vi "mxwScript_Cmnd2Str_startGeneration.vi"(8 "error in (no error)":errorcluster, 11 "data":variant) -> (0 "error out":errorcluster, 3 "outputString":string)   [LabVIEW 2020]
uses:
  codeGenAPISupport.llb/cgAPI_mxwScript_Cmnd_StartGenerationCommandData.ctl
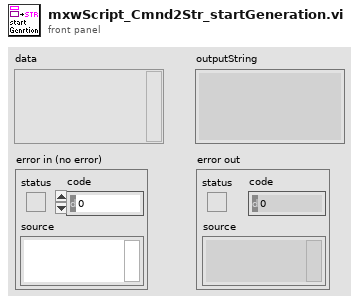
[diagram p1: front panel]
types:
  T1 = typedef "cgAPI_mxwScript_Cmnd_StartGenerationCommandData.ctl" = cluster{"VIref":refnum<vi>, "password":string}
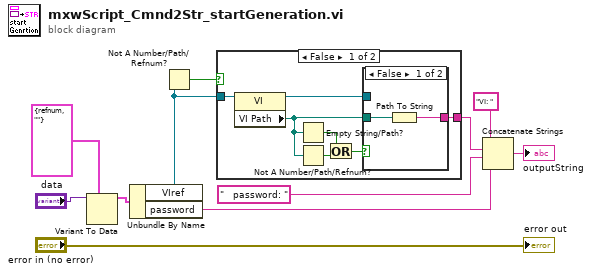
[diagram p0: block diagram]
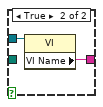
[diagram p2: hidden frame]
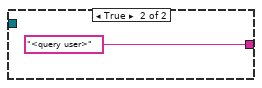
[diagram p3: hidden frame]
diagram:
  n1 = Variant To Data(type=T1 {"VIref"=refnum, "password"=""} ("vi refnum"), Variant="data") -> (data=w9:T1)  [unwired: 1 in, 1 out]
  n2 = Unbundle By Name(w9) -> ("VIref"=w7:refnum<vi>, "password"=w4:string)
  n3 = Not A Number/Path/Refnum?(number/path/refnum=w7) -> (NaN/Path/Refnum?=w8:bool)
  n4 = case shown="False" w8 {
    tunnel: w7 -> [w18 _]
    tunnel: [w13 "<query user>" ("Name")] -> w5
    frame False {
      n5 = property class="VI"(reference=w18) -> (reference out=w14:refnum<vi>, "VI Path"=w12:path)  [unwired: 1 in, 1 out]
      n6 = Empty String/Path?(string/path=w12) -> (empty?=w16:bool)
      n7 = Not A Number/Path/Refnum?(number/path/refnum=w12) -> (NaN/Path/Refnum?=w17:bool)
      n8 = Or(x=w16, y=w17) -> (x .or. y?=w15:bool)
      n9 = case shown="False" w15 {
        tunnel: w14 -> [_ w22]
        tunnel: [w19 w21] -> w13
        tunnel: w12 -> [w20 _]
        frame False {
          n10 = Path To String(path=w20) -> (string=w19:string)
        }
        frame True {
          n11 = property class="VI"(reference=w22) -> ("VI Name"=w21:string)  [unwired: 1 in, 2 out]
        }
      }
    }
    frame True {
    }
  }
  n12 = Concatenate Strings("VI: " ("Name"), w5, "   password: " ("Name"), w4) -> (→"outputString":string)
  "error out" <- "error in (no error)"
